vi "g_RobotMacros.vi"(7 "Action":enum16{"read", "write"}(ring), 10 "Macros":T1[](array[typedef]) {"Sequence"."Axes 2"."Switch" format="%#_4g"; "Sequence"."Axes 2"."Axis 2" format="%#_4g"; "Sequence"."Axes 2"."Axis 1" format="%#_4g"; "Sequence"."Axes 2"."Axis 0" format="%#_4g"; "Sequence"."Axes 1"."Axis 6" format="%#_4g"; "Sequence"."Axes 1"."Axis 5" format="%#_4g"; "Sequence"."Axes 1"."Axis 4" format="%#_4g"; "Sequence"."Axes 1"."Axis 3" format="%#_4g"; "Sequence"."Axes 1"."Axis 2" format="%#_4g"; "Sequence"."Axes 1"."Axis 1" format="%#_4g"}) -> (2 "Macros out":T1[](array[typedef]) {"Sequence"."Axes 2"."Switch" format="%#_4g"; "Sequence"."Axes 2"."Axis 2" format="%#_4g"; "Sequence"."Axes 2"."Axis 1" format="%#_4g"; "Sequence"."Axes 2"."Axis 0" format="%#_4g"; "Sequence"."Axes 1"."Axis 6" format="%#_4g"; "Sequence"."Axes 1"."Axis 5" format="%#_4g"; "Sequence"."Axes 1"."Axis 4" format="%#_4g"; "Sequence"."Axes 1"."Axis 3" format="%#_4g"; "Sequence"."Axes 1"."Axis 2" format="%#_4g"; "Sequence"."Axes 1"."Axis 1" format="%#_4g"})   [LabVIEW 2017]
uses:
  Ctrl Refs/Macros.ctl
  Ctrl Refs/JoyStick1.ctl
  Ctrl Refs/JoyStick1(Analog).ctl
  Ctrl Refs/JoyStick2.ctl
  Ctrl Refs/JoyStick2(Analog).ctl
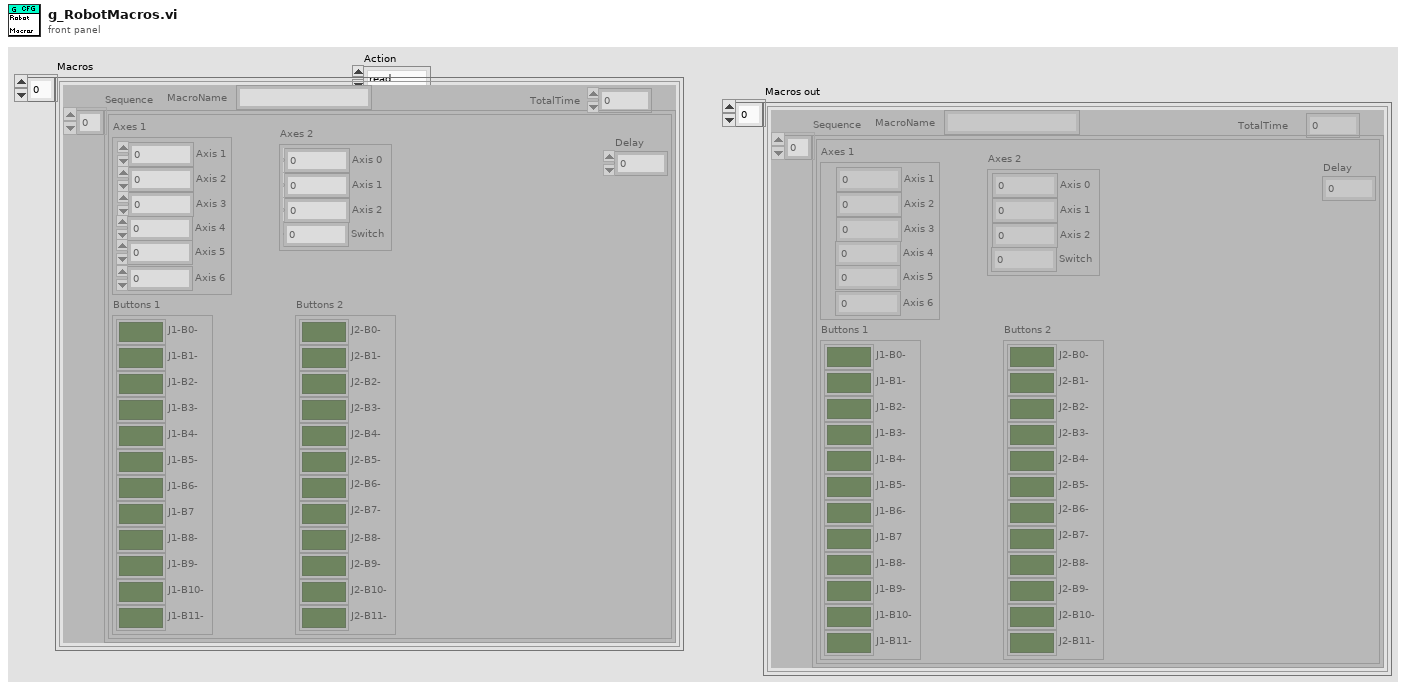
[diagram p1: front panel]
types:
  T1 = typedef "Macros.ctl" = cluster{"MacroName":string, "Sequence":cluster{"Buttons 1":T2, "Axes 1":T3, "Buttons 2":T4, "Axes 2":T5, "Delay":u32}[], "TotalTime":u32}
  T2 = typedef "JoyStick1.ctl" = cluster{"J1-B0-":bool, "J1-B1-":bool, "J1-B2-":bool, "J1-B3- ":bool, "J1-B4-":bool, "J1-B5-":bool, "J1-B6-":bool, "J1-B7":bool, "J1-B8-":bool, "J1-B9-":bool, "J1-B10-":bool, "J1-B11-":bool}
  T3 = typedef "JoyStick1(Analog).ctl" = cluster{"Axis 1":dbl, "Axis 2":dbl, "Axis 3":dbl, "Axis 4":dbl, "Axis 5":dbl, "Axis 6":dbl}
  T4 = typedef "JoyStick2.ctl" = cluster{"J2-B0-":bool, "J2-B1-":bool, "J2-B2-":bool, "J2-B3-":bool, "J2-B4-":bool, "J2-B5-":bool, "J2-B6-":bool, "J2-B7-":bool, "J2-B8-":bool, "J2-B9-":bool, "J2-B10-\n":bool, "J2-B11-":bool}
  T5 = typedef "JoyStick2(Analog).ctl" = cluster{"Axis 0":dbl, "Axis 1":dbl, "Axis 2":dbl, "Switch":dbl}
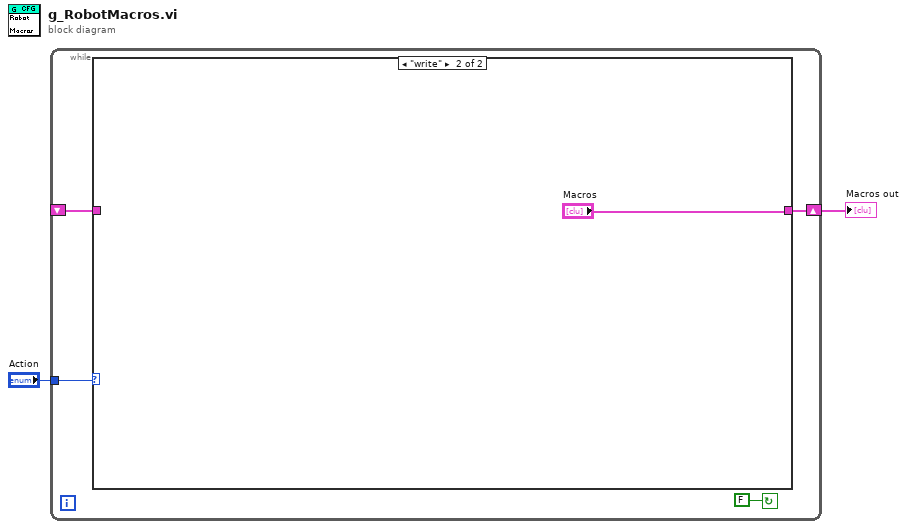
[diagram p0: block diagram]
diagram:
  n1 = while {
    tunnel: "Action" -> [w5]
    shift-right: [w4] -> w1
    shift-left: _ -> [w3]
    stop <- FALSE continue-if-true
    n2 = case shown="\"write\"" w5 {
      tunnel: [w7 "Macros"] -> w4
      tunnel: w3 -> [w7 _]
      frame "read", Default {
      }
      frame "write" {
      }
    }
  }
  "Macros out" <- w1
